vi "Lidar.vi"(1 "数值":i32, 2 "read buffer":string) -> (0 "输出簇":T1)   [LabVIEW 2014]
panel:
  out "16位整型 2":u16
  out "16位整型":u16
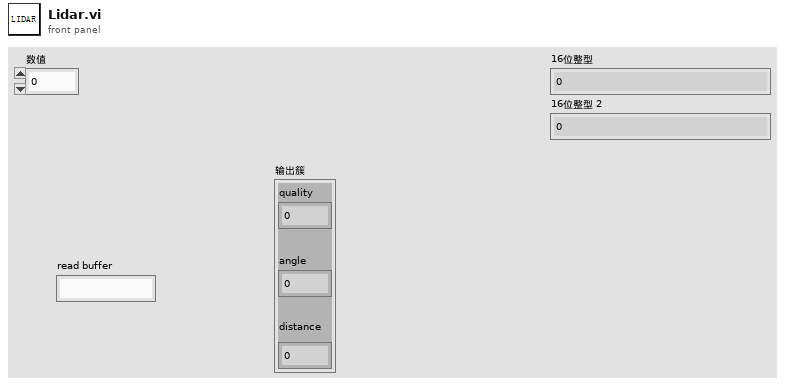
[diagram p1: front panel]
types:
  T1 = cluster{"quality":u8, "angle":u16, "distance\n":u16}
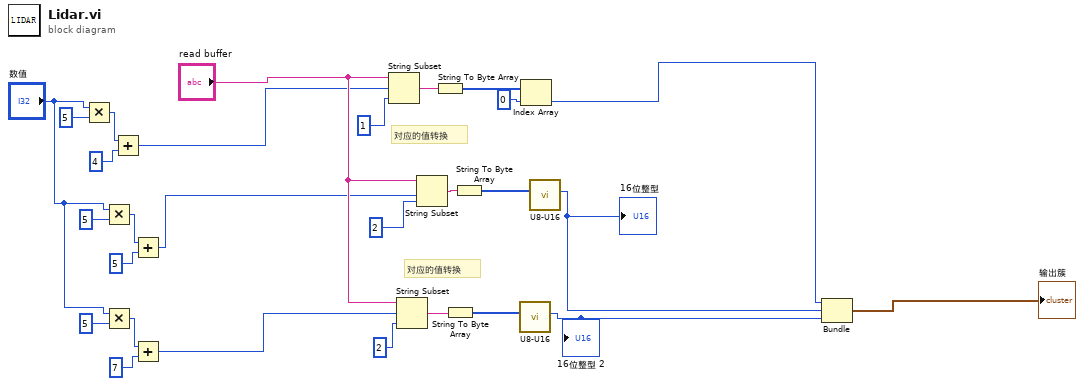
[diagram p0: block diagram]
diagram:
  # "对应的值转换"
  # "对应的值转换"
  n1 = Multiply(x="数值", y=u8 5) -> (x*y=w12:i32)
  n2 = Multiply(x="数值", y=u8 5) -> (x*y=w8:i32)
  n3 = Multiply(x="数值", y=u8 5) -> (x*y=w5:i32)
  n4 = Add(x=w12, y=4) -> (x+y=w10:i32)
  n5 = Add(x=w8, y=5) -> (x+y=w2:i32)
  n6 = Add(x=w5, y=7) -> (x+y=w1:i32)
  n7 = String Subset(string="read buffer", offset (0)=w10, length (rest)=1 ("长度（剩余）")) -> (substring=w26:string)
  n8 = String Subset(string="read buffer", offset (0)=w1, length (rest)=2 ("长度（剩余）")) -> (substring=w28:string)
  n9 = String Subset(string="read buffer", offset (0)=w2, length (rest)=2 ("长度（剩余）")) -> (substring=w19:string)
  n10 = String To Byte Array(string=w26) -> (unsigned byte array=w23:u8[])
  n11 = String To Byte Array(string=w28) -> (unsigned byte array=w20:u8[])
  n12 = String To Byte Array(string=w19) -> (unsigned byte array=w15:u8[])
  n13 = call "U8-U16.vi"("数组"=w20) -> ("16位整型"=w16:u16)  [unwired: 8 in, 1 out]
  "16位整型 2" <- w16
  n14 = Index Array(array=w23, index=0 ("索引")) -> (element=w21:u8)
  n15 = call "U8-U16.vi"("数组"=w15) -> ("16位整型"=w14:u16)  [unwired: 8 in, 1 out]
  "16位整型" <- w14
  n16 = Bundle(w21, "16位整型"=w14, "16位整型"=w16) -> (→"输出簇":cluster{u8, "16位整型":u16, "16位整型":u16})  [unwired: 1 in]
